vi "DCP Config.vi"(8 "error in (no error)":errorcluster, 11 "Device Reference In":T1 format="%.0x") -> (0 "error out":errorcluster, 1 "Limit Behaviour":u16[](array[numeric]), 2 "Channels":string[](array[string]), 3 "instrument handle out":refnum<k15>)   [LabVIEW 2011, in "IVI DC Power Supply Custom Device.lvlib"]
uses:
  IVI DC Power Supply Custom Device.lvlib
  <vilib>/NI Veristand/Custom Device API/Custom Device Item Ref.ctl
  Global.vi
  <vilib>/NI Veristand/Custom Device API/Get Item Property (String).vi
  <vilib>/NI Veristand/Custom Device Tools/Custom Device Utility Library/NI VeriStand - Search for All Items by GUID.vi
  <vilib>/NI Veristand/Custom Device API/Get Item Property (U16).vi
  <vilib>/NI Veristand/Custom Device API/Get Item Property (Boolean).vi
  <vilib>/NI Veristand/Custom Device API/Get Item Property (Double).vi
  <vilib>/NI Veristand/Custom Device API/Custom Device API.lvlib
  <vilib>/NI Veristand/Custom Device Tools/Custom Device Utility Library/Custom Device Utility Library.lvlib
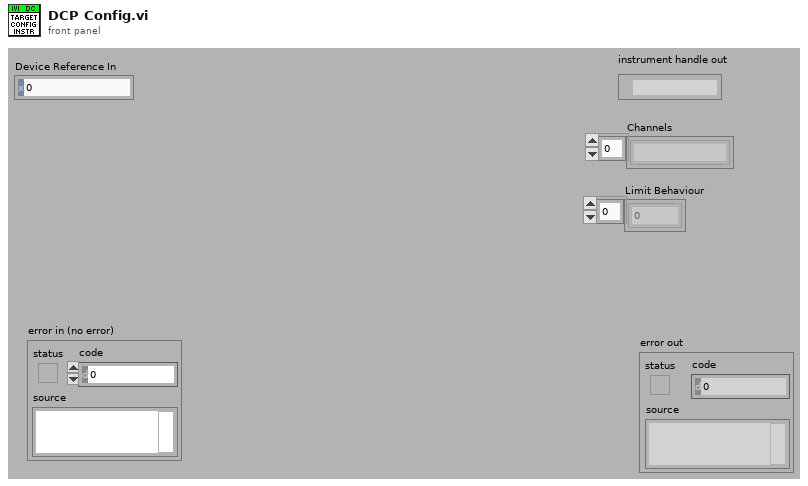
[diagram p1: front panel]
types:
  T1 = typedef "Custom Device API.lvlib/Custom Device Item Ref.ctl" = u64
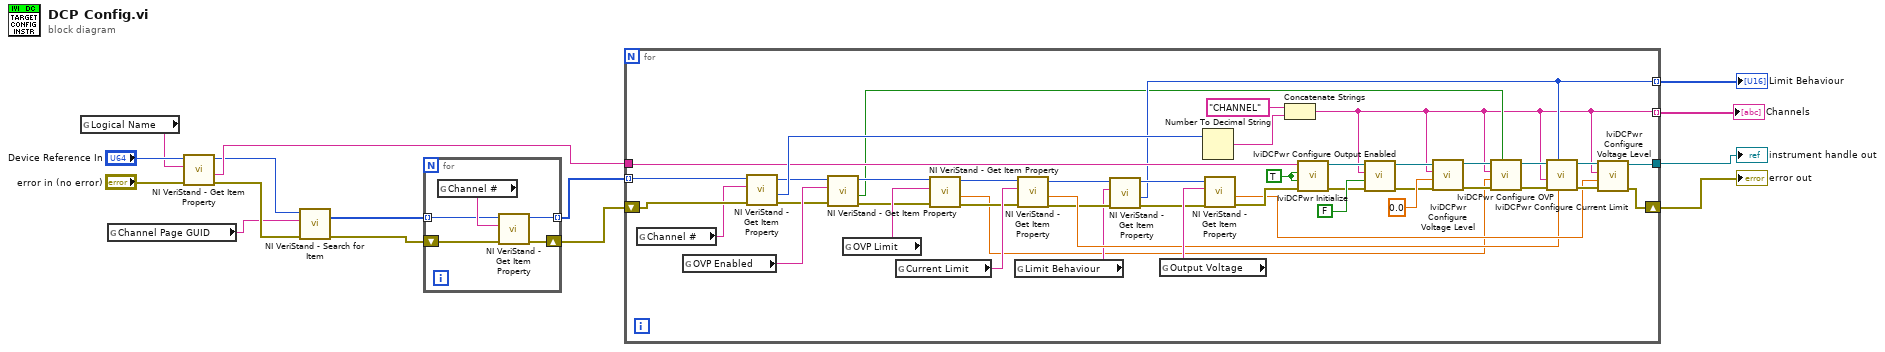
[diagram p0: block diagram]
diagram:
  n1 = global read "Global.vi" "Logical Name"() -> (w9:string)
  n2 = global read "Global.vi" "Channel Page GUID"() -> (w3:string)
  n3 = call-poly <vilib>:"NI VeriStand - Get Item Property.vi"("error in (no error)"="error in (no error)", "Property Name"=w9, "Item Ref in"="Device Reference In") -> ("error out"=w4:errorcluster, "Value"=w10:string, "Item Ref out"=w5:T1)  [unwired: 5 in, 1 out]
  n4 = call-poly <vilib>:"NI VeriStand - Search for Item.vi"("error in"=w4, "Item GUID"=w3, "Section Ref in"=w5) -> ("error out"=w2:errorcluster, "Item Refs"=w6:T1[])  [unwired: 5 in, 2 out]
  n5 = for {
    tunnel: w6 -> [w17] mode=indexing
    shift-right: [w18] -> w8
    shift-left: w2 -> [w19]
    tunnel: [w16] -> w1 mode=indexing
    n6 = global read "Global.vi" "Channel #"() -> (w20:string)
    n7 = call-poly <vilib>:"NI VeriStand - Get Item Property.vi"("error in (no error)"=w19, "Property Name"=w20, "Item Ref in"=w17) -> ("error out"=w18:errorcluster, "Item Ref out"=w16:T1)  [unwired: 5 in, 2 out]
  }
  n8 = for {
    tunnel: [w49] -> w13
    tunnel: w10 -> [w52]
    shift-right: [w48] -> w12
    shift-left: w8 -> [w64]
    tunnel: [w23] -> w11 mode=indexing
    tunnel: [w37] -> w7 mode=indexing
    tunnel: w1 -> [w21] mode=indexing
    w53 = TRUE ("id query (True)")
    n9 = global read "Global.vi" "Channel #"() -> (w63:string)
    n10 = global read "Global.vi" "OVP Enabled"() -> (w32:string)
    n11 = call-poly <vilib>:"NI VeriStand - Get Item Property.vi"("error in (no error)"=w64, "Property Name"=w63, "Item Ref in"=w21) -> ("error out"=w27:errorcluster, "Value"=w61:u16, "Item Ref out"=w31:T1)  [unwired: 5 in, 1 out]
    n12 = call-poly <vilib>:"NI VeriStand - Get Item Property.vi"("error in (no error)"=w27, "Property Name"=w32, "Item Ref in"=w31) -> ("error out"=w26:errorcluster, "Value"=w24:bool, "Item Ref out"=w30:T1)  [unwired: 5 in, 1 out]
    n13 = global read "Global.vi" "OVP Limit"() -> (w28:string)
    n14 = global read "Global.vi" "Current Limit"() -> (w47:string)
    n15 = call-poly <vilib>:"NI VeriStand - Get Item Property.vi"("error in (no error)"=w26, "Property Name"=w28, "Item Ref in"=w30) -> ("error out"=w25:errorcluster, "Value"=w22:dbl, "Item Ref out"=w29:T1)  [unwired: 5 in, 1 out]
    n16 = global read "Global.vi" "Limit Behaviour"() -> (w38:string)
    n17 = call-poly <vilib>:"NI VeriStand - Get Item Property.vi"("error in (no error)"=w25, "Property Name"=w47, "Item Ref in"=w29) -> ("error out"=w40:errorcluster, "Value"=w43:dbl, "Item Ref out"=w42:T1)  [unwired: 5 in, 1 out]
    n18 = call-poly <vilib>:"NI VeriStand - Get Item Property.vi"("error in (no error)"=w40, "Property Name"=w38, "Item Ref in"=w42) -> ("error out"=w39:errorcluster, "Value"=w37:u16, "Item Ref out"=w41:T1)  [unwired: 5 in, 1 out]
    n19 = global read "Global.vi" "Output Voltage"() -> (w46:string)
    n20 = Number To Decimal String(number=w61) -> (decimal integer string=w60:string)  [unwired: 1 in]
    n21 = call-poly <vilib>:"NI VeriStand - Get Item Property.vi"("error in (no error)"=w39, "Property Name"=w46, "Item Ref in"=w41) -> ("error out"=w45:errorcluster, "Value"=w44:dbl)  [unwired: 5 in, 2 out]
    n22 = Concatenate Strings("CHANNEL" ("string"), w60) -> (w23:string)
    n23 = call <vilib>:"IviDCPwr Initialize.vi"("error in (no error)"=w45, "reset device (True)"=w53, "id query (True)"=w53, "logical name (\"SamplePowerSupply\")"=w52) -> ("error out"=w54:errorcluster, "instrument handle"=w56:refnum<k15>)  [unwired: 6 in]
    n24 = call <vilib>:"IviDCPwr Configure Output Enabled.vi"("error in (no error)"=w54, "enabled (true)"=FALSE, "channel name (\"CHANNEL1\")"=w23, "instrument handle"=w56) -> ("error out"=w57:errorcluster, "instrument handle out"=w59:refnum<k15>)  [unwired: 6 in]
    n25 = call <vilib>:"IviDCPwr Configure Voltage Level.vi"("error in (no error)"=w57, "level (0.0 Volts)"=0.0, "channel name (\"CHANNEL1\")"=w23, "instrument handle"=w59) -> ("error out"=w36:errorcluster, "instrument handle out"=w35:refnum<k15>)  [unwired: 6 in]
    n26 = call <vilib>:"IviDCPwr Configure OVP.vi"("enabled (true)"=w24, "error in (no error)"=w36, "limit (0.0 Volts)"=w22, "channel name (\"CHANNEL1\")"=w23, "instrument handle"=w35) -> ("error out"=w34:errorcluster, "instrument handle out"=w33:refnum<k15>)  [unwired: 5 out]
    n27 = call <vilib>:"IviDCPwr Configure Current Limit.vi"("limit (0.0 Amps)"=w43, "behavior (regulate)"=w37, "error in (no error)"=w34, "channel name (\"CHANNEL1\")"=w23, "instrument handle"=w33) -> ("error out"=w51:errorcluster, "instrument handle out"=w50:refnum<k15>)  [unwired: 5 out]
    n28 = call <vilib>:"IviDCPwr Configure Voltage Level.vi"("error in (no error)"=w51, "level (0.0 Volts)"=w44, "channel name (\"CHANNEL1\")"=w23, "instrument handle"=w50) -> ("error out"=w48:errorcluster, "instrument handle out"=w49:refnum<k15>)  [unwired: 6 out]
  }
  "error out" <- w12
  "instrument handle out" <- w13
  "Channels" <- w11
  "Limit Behaviour" <- w7
